vi "Configure.vi"   [LabVIEW 2021, in "AudioGeneration.lvclass"]
uses:
  AudioGeneration.lvclass
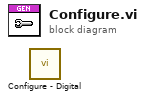
[diagram p0: block diagram]
diagram:
  n1 = call "Configure - Digital.vi"() -> ()  [unwired: 10 in, 2 out]
